vi "add action dialog.vi"(8 "error in (no error)":errorcluster, 11 "supported actions list":T1[](array[typedef])) -> (0 "error out":errorcluster, 2 "cancelled":bool, 3 "config and UI pairing":T1)   [LabVIEW 2014, in "Simple Sequencer TBM editor node.lvclass"]
doc: "Displays a dialog that allows a uers to specify which action they would like to add to a sequence."
uses:
  Simple Sequencer TBM editor node.lvclass
  action config and UI pairing.ctl
  sequencer parent classes/action configuration parent/action configuration.lvclass
panel:
  in  "cancel":bool
  in  "OK":bool
  in  "Available Actions":i32(listbox)
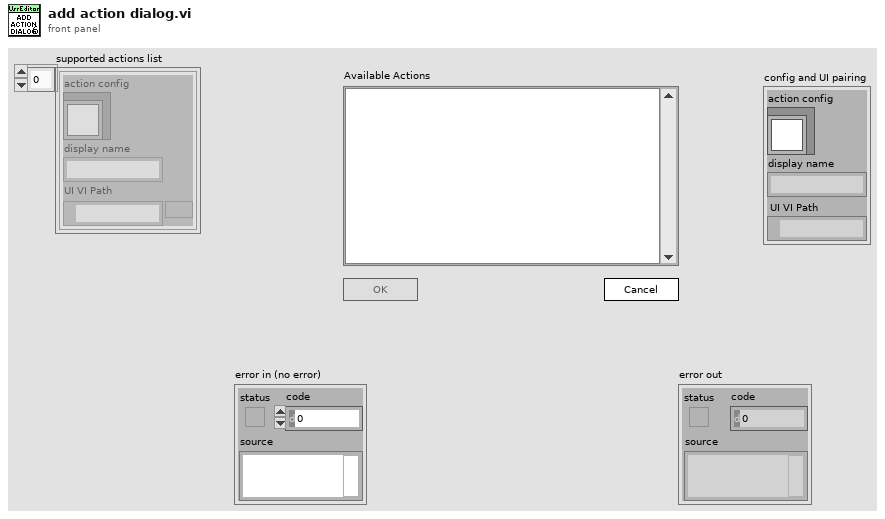
[diagram p1: front panel]
types:
  T1 = typedef "Simple Sequencer TBM editor node.lvclass/action config and UI pairing.ctl" = cluster{"action config":refnum<class "action configuration.lvclass">, "display name":string, "UI VI Path":path}
  T2 = enum8{"Enabled", "Disabled", "Disabled and Grayed Out"}
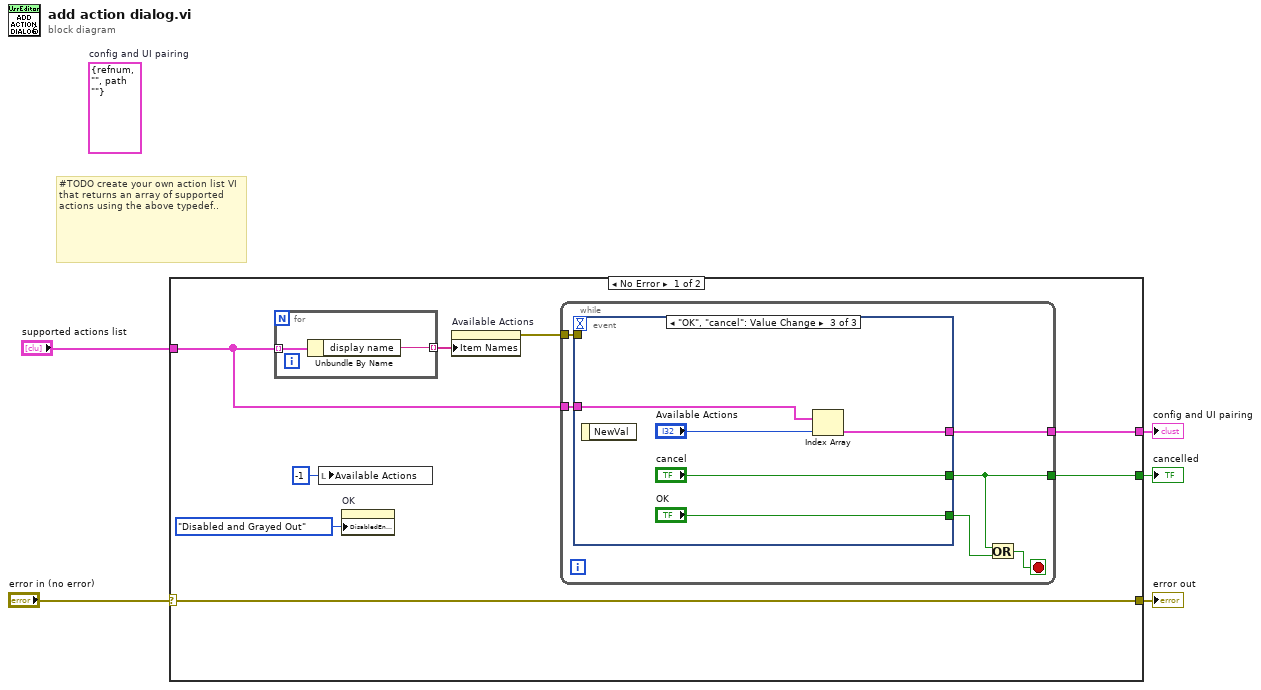
[diagram p0: block diagram]
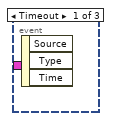
[diagram p2: hidden frame]
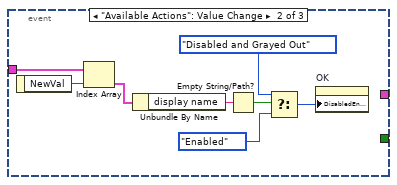
[diagram p3: hidden frame]
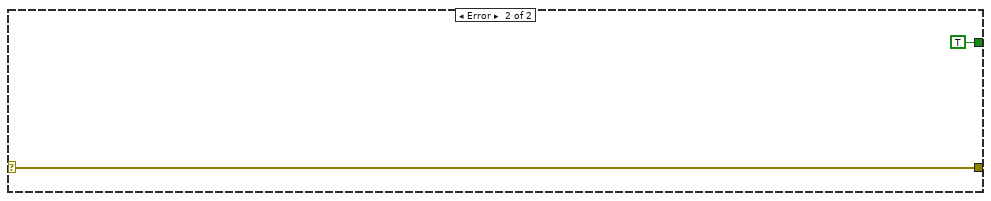
[diagram p4: hidden frame]
diagram:
  (unwired) T1 {"action config"=refnum, "display name"="", "UI VI Path"=path ""}  # config and UI pairing
  # "#TODO create your own action list VI that returns an array of supported actions using the above typedef.."
  n1 = case shown="No Error" "error in (no error)" {
    selector: "error in (no error)" -> [w13 w36]
    tunnel: [w13 w36] -> w5
    tunnel: "supported actions list" -> [w7 _]
    tunnel: [w9 TRUE ("cancel")] -> w4
    tunnel: [w8 _] -> w3
    frame No Error {
      n2 = for {
        tunnel: w7 -> [w34] mode=indexing
        tunnel: [w33] -> w11 mode=indexing
        n3 = Unbundle By Name(w34) -> ("display name"=w33:string)
      }
      n4 = local write "Available Actions"(-1 ("Available Actions")) -> ()
      n5 = property on="OK" class="Bool"("DisabledEnum"=T2."Disabled and Grayed Out" ("Disabled")) -> ()  [unwired: 2 in, 2 out]
      n6 = property on="Available Actions" class="LstBox (strict)"("Item Names"=w11) -> (error out=w12:errorcluster)  [unwired: 2 in, 1 out]
      n7 = while {
        tunnel: w12 -> [w19]
        tunnel: w7 -> [w18]
        tunnel: [w16] -> w9
        tunnel: [w14] -> w8
        stop <- w15 stop-if-true
        n8 = event shown="[2] \"OK\", \"cancel\": Value Change" {
          selector: _ -> [_ _ _]
          dyn-events: _ -> [_ _ _]
          timeout: _ -> [_ _ _]
          tunnel: w19 -> [_ _ _]
          tunnel: w18 -> [_ w22 w29]
          tunnel: [_ _ "OK"] -> w17
          tunnel: [_ _ "cancel"] -> w16
          tunnel: [_ _ w28] -> w14
          event Timeout {
            n9 = event-data() -> ()  [unwired: 1 in, 3 out]
          }
          event "Available Actions": Value Change {
            n10 = event-data() -> ("NewVal"=w27:i32)  [unwired: 1 in]
            n11 = Index Array(array=w22, index=w27) -> (element=w21:T1)
            n12 = Unbundle By Name(w21) -> ("display name"=w20:string)
            n13 = Empty String/Path?(string/path=w20) -> (empty?=w26:bool)
            n14 = Select(t=T2."Disabled and Grayed Out" ("Disabled"), s=w26, f=T2."Enabled" ("Disabled")) -> (s? t:f=w23:T2)
            n15 = property on="OK" class="Bool"("DisabledEnum"=w23) -> ()  [unwired: 2 in, 2 out]
          }
          event "OK", "cancel": Value Change {
            n16 = event-data() -> ()  [unwired: 1 in, 1 out]
            n17 = Index Array(array=w29, index="Available Actions") -> (element=w28:T1)
          }
        }
        n18 = Or(x=w16, y=w17) -> (x .or. y?=w15:bool)
      }
    }
    frame Error {
    }
  }
  "error out" <- w5
  "cancelled" <- w4
  "config and UI pairing" <- w3
